vi "Rolling Display.vi"(6 "Input Data":dbl[][](array[numeric]), 8 "Channels in Use":T2, 9 "Old Data":dbl[][](array[numeric]), 10 "Sample Rate":i32, 11 "Display Size":T3(ring)) -> (1 "Output Array Values":dbl[][](array[numeric]), 3 "Output Waveform Cluster":T1)   [LabVIEW 2014]
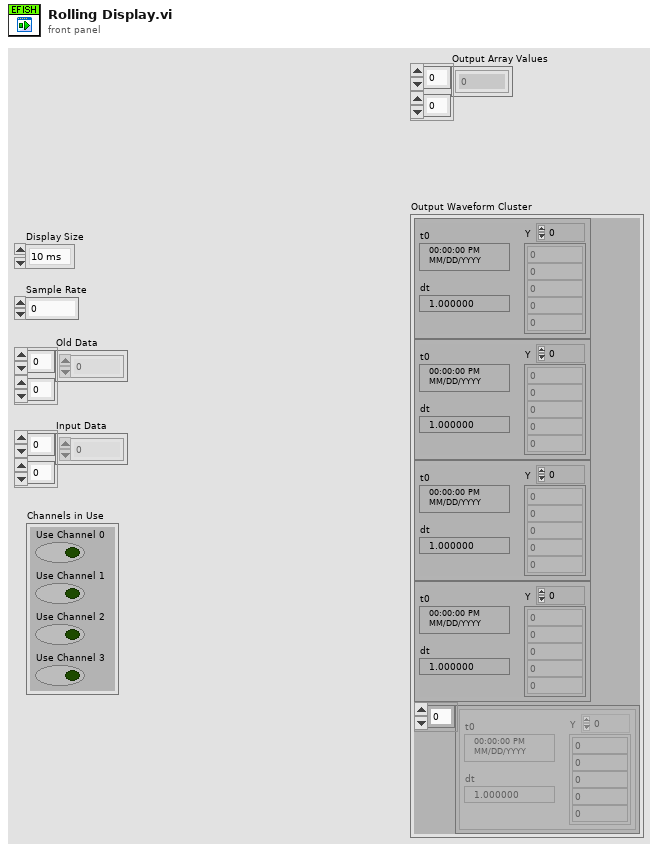
[diagram p1: front panel]
types:
  T1 = cluster{"Waveform":waveform(dbl), "Waveform":waveform(dbl), "Waveform":waveform(dbl), "Waveform":waveform(dbl), waveform(dbl)[]}
  T2 = cluster{"Use Channel 0":bool, "Use Channel 1":bool, "Use Channel 2":bool, "Use Channel 3":bool}
  T3 = enum16{"10 ms", "100 ms", "1 Second", "10 sec", "30 sec"}
  T4 = cluster{waveform(dbl), waveform(dbl), waveform(dbl), waveform(dbl), waveform(dbl)[]}
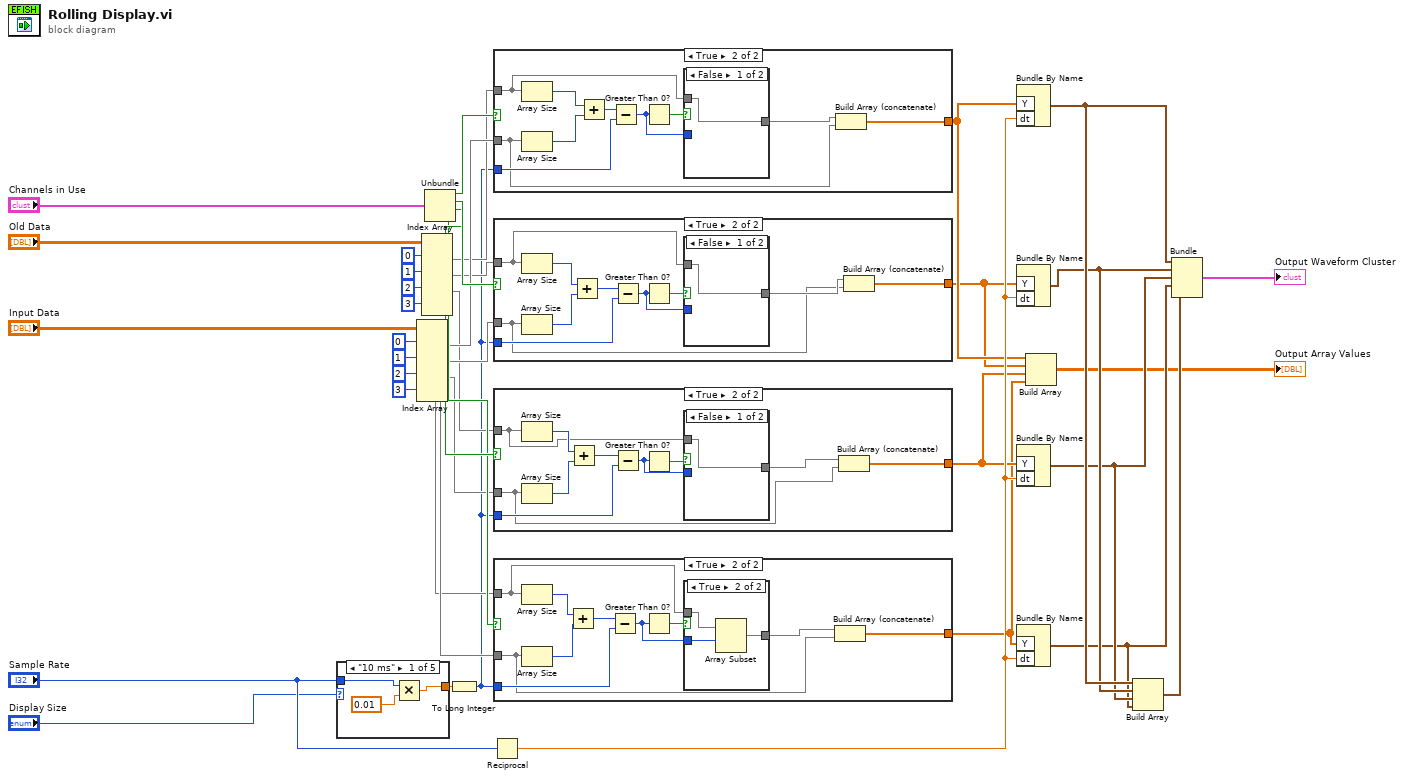
[diagram p0: block diagram]
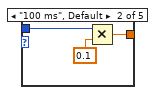
[diagram p2: hidden frame]
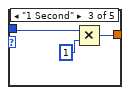
[diagram p3: hidden frame]
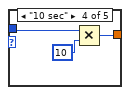
[diagram p4: hidden frame]
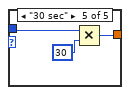
[diagram p5: hidden frame]
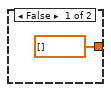
[diagram p6: hidden frame]
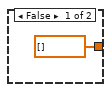
[diagram p8: hidden frame]
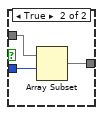
[diagram p9: hidden frame]
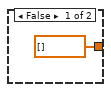
[diagram p10: hidden frame]
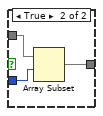
[diagram p11: hidden frame]
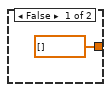
[diagram p12: hidden frame]
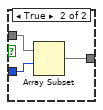
[diagram p13: hidden frame]
diagram:
  n1 = case shown="\"10 ms\"" "Display Size" {
    tunnel: "Sample Rate" -> [w41 w45 w47 w50 w53]
    tunnel: [w42 w43 w48 w51 w54] -> w17
    frame "10 ms" {
      n2 = Multiply(x=w41, y=0.01) -> (x*y=w42:dbl)
    }
    frame "100 ms", Default {
      n3 = Multiply(x=w45, y=0.1) -> (x*y=w43:dbl)
    }
    frame "1 Second" {
      n4 = Multiply(x=w47, y=1) -> (x*y=w48:i32)
    }
    frame "10 sec" {
      n5 = Multiply(x=w50, y=10) -> (x*y=w51:i32)
    }
    frame "30 sec" {
      n6 = Multiply(x=w53, y=30) -> (x*y=w54:i32)
    }
  }
  n7 = Index Array(array="Input Data", index (row) #1=0 ("index (row)"), index (row) #2=1 ("index (row)"), index (row) #3=2 ("index (row)"), index (row) #4=3 ("index (row)")) -> (element #1=w26:dbl[], element #2=w25:dbl[], element #3=w24:dbl[], element #4=w23:dbl[])  [unwired: 4 in]
  n8 = Index Array(array="Old Data", index (row) #1=0 ("index (row)"), index (row) #2=1 ("index (row)"), index (row) #3=2 ("index (row)"), index (row) #4=3 ("index (row)")) -> (element #1=w21:dbl[], element #2=w20:dbl[], element #3=w19:dbl[], element #4=w18:dbl[])  [unwired: 4 in]
  n9 = Unbundle("Channels in Use") -> ("Use Channel 0"=w34:bool, "Use Channel 1"=w33:bool, "Use Channel 2"=w32:bool, "Use Channel 3"=w31:bool)
  n10 = To Long Integer(number=w17) -> (32bit integer=w16:i32)
  n11 = Reciprocal(x="Sample Rate") -> (1/x=w15:dbl)
  n12 = case shown="True" w34 {
    tunnel: w26 -> [_ w56]
    tunnel: w21 -> [_ w59]
    tunnel: w16 -> [_ w62]
    tunnel: [dbl[] [] w58] -> w9
    frame False {
    }
    frame True {
      n13 = Array Size(array=w59) -> (size(s)=w65:i32)
      n14 = Array Size(array=w56) -> (size(s)=w64:i32)
      n15 = Add(x=w65, y=w64) -> (x+y=w63:i32)
      n16 = Subtract(x=w63, y=w62) -> (x-y=w60:i32)
      n17 = Greater Than 0?(x=w60) -> (x > 0?=w61:bool)
      n18 = case shown="False" w61 {
        tunnel: w60 -> [_ w69]
        tunnel: w59 -> [w66 w68]
        tunnel: [w66 w67] -> w57
        frame False {
        }
        frame True {
          n19 = Array Subset(array=w68, index=w69) -> (w67:dbl[])  [unwired: 1 in]
        }
      }
      n20 = Build Array (concatenate)(w57, w56) -> (w58:dbl[])
    }
  }
  n21 = case shown="True" w33 {
    tunnel: w25 -> [_ w71]
    tunnel: w20 -> [_ w74]
    tunnel: w16 -> [_ w77]
    tunnel: [dbl[] [] w73] -> w8
    frame False {
    }
    frame True {
      n22 = Array Size(array=w74) -> (size(s)=w80:i32)
      n23 = Array Size(array=w71) -> (size(s)=w79:i32)
      n24 = Add(x=w80, y=w79) -> (x+y=w78:i32)
      n25 = Subtract(x=w78, y=w77) -> (x-y=w75:i32)
      n26 = Greater Than 0?(x=w75) -> (x > 0?=w76:bool)
      n27 = case shown="False" w76 {
        tunnel: w75 -> [_ w84]
        tunnel: w74 -> [w81 w83]
        tunnel: [w81 w82] -> w72
        frame False {
        }
        frame True {
          n28 = Array Subset(array=w83, index=w84) -> (w82:dbl[])  [unwired: 1 in]
        }
      }
      n29 = Build Array (concatenate)(w72, w71) -> (w73:dbl[])
    }
  }
  n30 = case shown="True" w32 {
    tunnel: w24 -> [_ w86]
    tunnel: w19 -> [_ w89]
    tunnel: w16 -> [_ w92]
    tunnel: [dbl[] [] w88] -> w7
    frame False {
    }
    frame True {
      n31 = Array Size(array=w89) -> (size(s)=w95:i32)
      n32 = Array Size(array=w86) -> (size(s)=w94:i32)
      n33 = Add(x=w95, y=w94) -> (x+y=w93:i32)
      n34 = Subtract(x=w93, y=w92) -> (x-y=w90:i32)
      n35 = Greater Than 0?(x=w90) -> (x > 0?=w91:bool)
      n36 = case shown="False" w91 {
        tunnel: w90 -> [_ w99]
        tunnel: w89 -> [w96 w98]
        tunnel: [w96 w97] -> w87
        frame False {
        }
        frame True {
          n37 = Array Subset(array=w98, index=w99) -> (w97:dbl[])  [unwired: 1 in]
        }
      }
      n38 = Build Array (concatenate)(w87, w86) -> (w88:dbl[])
    }
  }
  n39 = case shown="True" w31 {
    tunnel: w23 -> [_ w102]
    tunnel: w18 -> [_ w104]
    tunnel: w16 -> [_ w107]
    tunnel: [dbl[] [] w103] -> w6
    frame False {
    }
    frame True {
      n40 = Array Size(array=w104) -> (size(s)=w110:i32)
      n41 = Array Size(array=w102) -> (size(s)=w109:i32)
      n42 = Add(x=w110, y=w109) -> (x+y=w108:i32)
      n43 = Subtract(x=w108, y=w107) -> (x-y=w105:i32)
      n44 = Greater Than 0?(x=w105) -> (x > 0?=w106:bool)
      n45 = case shown="True" w106 {
        tunnel: w105 -> [_ w114]
        tunnel: w104 -> [w111 w113]
        tunnel: [w111 w112] -> w101
        frame False {
        }
        frame True {
          n46 = Array Subset(array=w113, index=w114) -> (w112:dbl[])  [unwired: 1 in]
        }
      }
      n47 = Build Array (concatenate)(w101, w102) -> (w103:dbl[])
    }
  }
  n48 = Bundle By Name("Y"=w9, "dt"=w15) -> (w14:waveform(dbl))  [unwired: 1 in]
  n49 = Bundle By Name("Y"=w8, "dt"=w15) -> (w13:waveform(dbl))  [unwired: 1 in]
  n50 = Bundle By Name("Y"=w7, "dt"=w15) -> (w12:waveform(dbl))  [unwired: 1 in]
  n51 = Bundle By Name("Y"=w6, "dt"=w15) -> (w11:waveform(dbl))  [unwired: 1 in]
  n52 = Build Array(w9, w8, w7, w6) -> (→"Output Array Values":dbl[][])
  n53 = Build Array(w14, w13, w12, w11) -> (w10:waveform(dbl)[])
  n54 = Bundle(w14, w13, w12, w11, w10) -> (→"Output Waveform Cluster":T4)  [unwired: 1 in]
